vi "Comparison of the K-Means and MiniBatchKMeans clustering.vi"() -> ()   [LabVIEW 2020]
doc: "We want to compare the performance of the MiniBatchKMeans and KMeans: the MiniBatchKMeans is faster, but gives slightly different results.\n\nWe will cluster a set of data, first with KMeans and then with MiniBatchKMeans, and plot the results. We will also plot the points that are labelled differently between the two algorithms."
uses:
  Model/Unsupervised/Cluster/KMeans/Controls/kmeans_params.ctl
  Model/Unsupervised/Cluster/MiniBatchKMeans/Controls/mini_batch_kmeans_params.ctl
  PLAIYDISPLAY/Display/Classification/2D/Predicted/Controls/PredictedParameter.ctl
  PLAIYDISPLAY/Display/_Controls/Style.ctl
  Model/Unsupervised/Cluster/KMeans/KMeans.lvclass
  C:/Users/cipop/TDF Dropbox/2_Technologies de France/1 - Services et Etudes/PLAIY/2 - DEV/PLAIYLAB/code/Model/Model.lvclass
  Model/Unsupervised/Cluster/MiniBatchKMeans/MiniBatchKMeans.lvclass
  Model/Unsupervised/Cluster/KMeans/KMeans.vi
  Model/Unsupervised/Cluster/MiniBatchKMeans/MiniBatchKMeans.vi
  Preproc/Objet/6 - Datasets Transformation/6.8 - Pairwise metrics, Affinities and Kernels/Pairwise_distances_argmin/Pairwise_Distances_Argmin.vi
panel:
  in  "error in (no error)":errorcluster caption="entrée d'erreur (pas d'erreur)"
  in  "Local":T1
  out "identic":bool[](array[boolean])
  out "different":bool[](array[boolean])
  out "n_clusters":i32
  out "Plot 3":cluster{"X":dbl[], "Y":dbl[]}[](graph) caption="Difference"
  out "Plot 2":cluster{"X":dbl[], "Y":dbl[]}[](graph) caption="MiniBatchKMeans"
  out "error out":errorcluster
  out "Plot":cluster{"X":dbl[], "Y":dbl[]}[](graph) caption="KMeans"
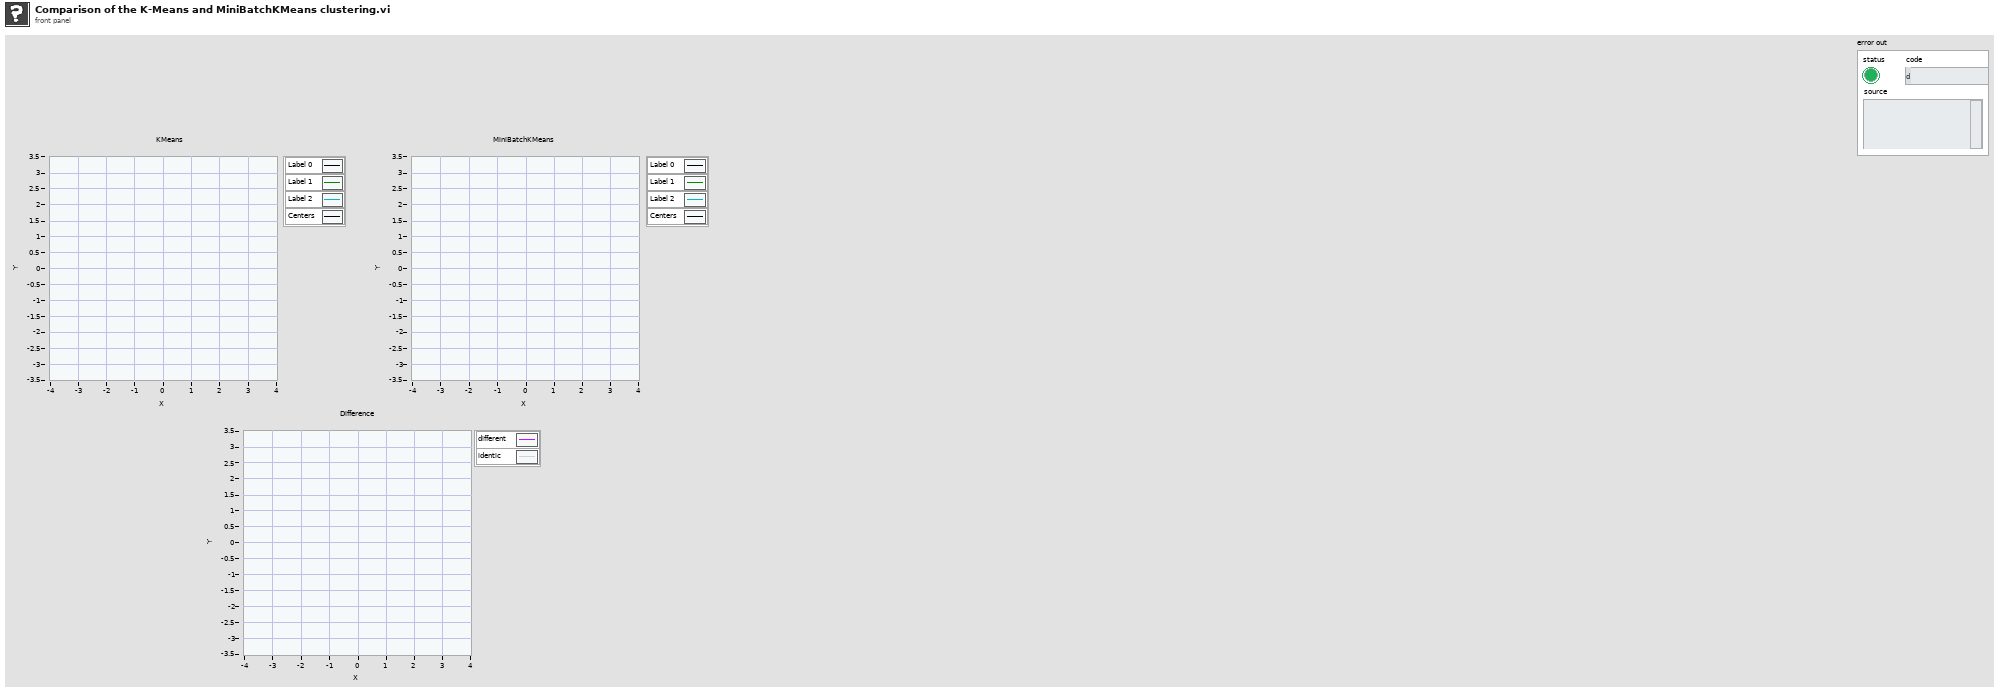
[diagram p1: front panel]
types:
  T1 = cluster{"X":dbl[][], "k_means_cluster_centers":dbl[][], "mbk.cluster_centers_":dbl[][], "k_means_labels":dbl[], "mbk_means_labels":dbl[], "order":dbl[], "mbk_means_cluster_centers":dbl[][]}
  T2 = cluster{"n_samples":i32[], "n_features":u32, "centers":i32[][], "cluster_std":dbl[], "centermin":dbl, "centermax":dbl, "shuffle":bool, "random_state":i32, "Returns":string}
  T3 = typedef "kmeans_params.ctl" = cluster{"n_clusters":dbl, "init":cluster{"init_type":string, "init_list":dbl[][]}, "n_init":dbl, "max_iter":dbl, "tol":dbl, "verbose":dbl, "random_state":dbl, "copy_x":bool, "algorithm":string}
  T4 = typedef "mini_batch_kmeans_params.ctl" = cluster{"n_clusters":dbl, "init":cluster{"init_type":string, "init_list":dbl[][]}, "max_iter":dbl, "batch_size":dbl, "verbose":dbl, "compute_labels":bool, "random_state":dbl, "tol":dbl, "max_no_improvement":dbl, "init_size":cluster{"init_size_type":string, "init_size_int":dbl}, "n_init":dbl, "reassignment_ratio":dbl}
  T5 = typedef "Style.ctl" = enum16{"Empty circle", "Full circle", "Empty square", "Full square", "Cross"}
  T6 = typedef "PredictedParameter.ctl" = cluster{"Plot":refnum<vi>, "Data":cluster{"X":dbl[][], "Predict":dbl[][]}, "Indexe":cluster{"X":i32, "Y":i32}, "Point Property":cluster{"Style":T5, "Label Color":u32[]}}
  T7 = cluster{" 4DArray":cluster{"1":string[][], "2":string[][]}[], " 3DArray":cluster{"Tableau":string[][]}[], "Sparse Matrix 2DArray":string[][], " 2DArray":string[][], " 1DArray":string[]}
  T8 = typedef "kmeans_attributes.ctl" = cluster{"cluster_centers_":dbl[][], "labels_":dbl[], "inertia_":dbl, "n_iter_":dbl}
  T9 = typedef "mini_batch_kmeans_attributes.ctl" = cluster{"cluster_centers_":dbl[][], "labels_":dbl[], "inertia_":dbl, "n_iter_":dbl}
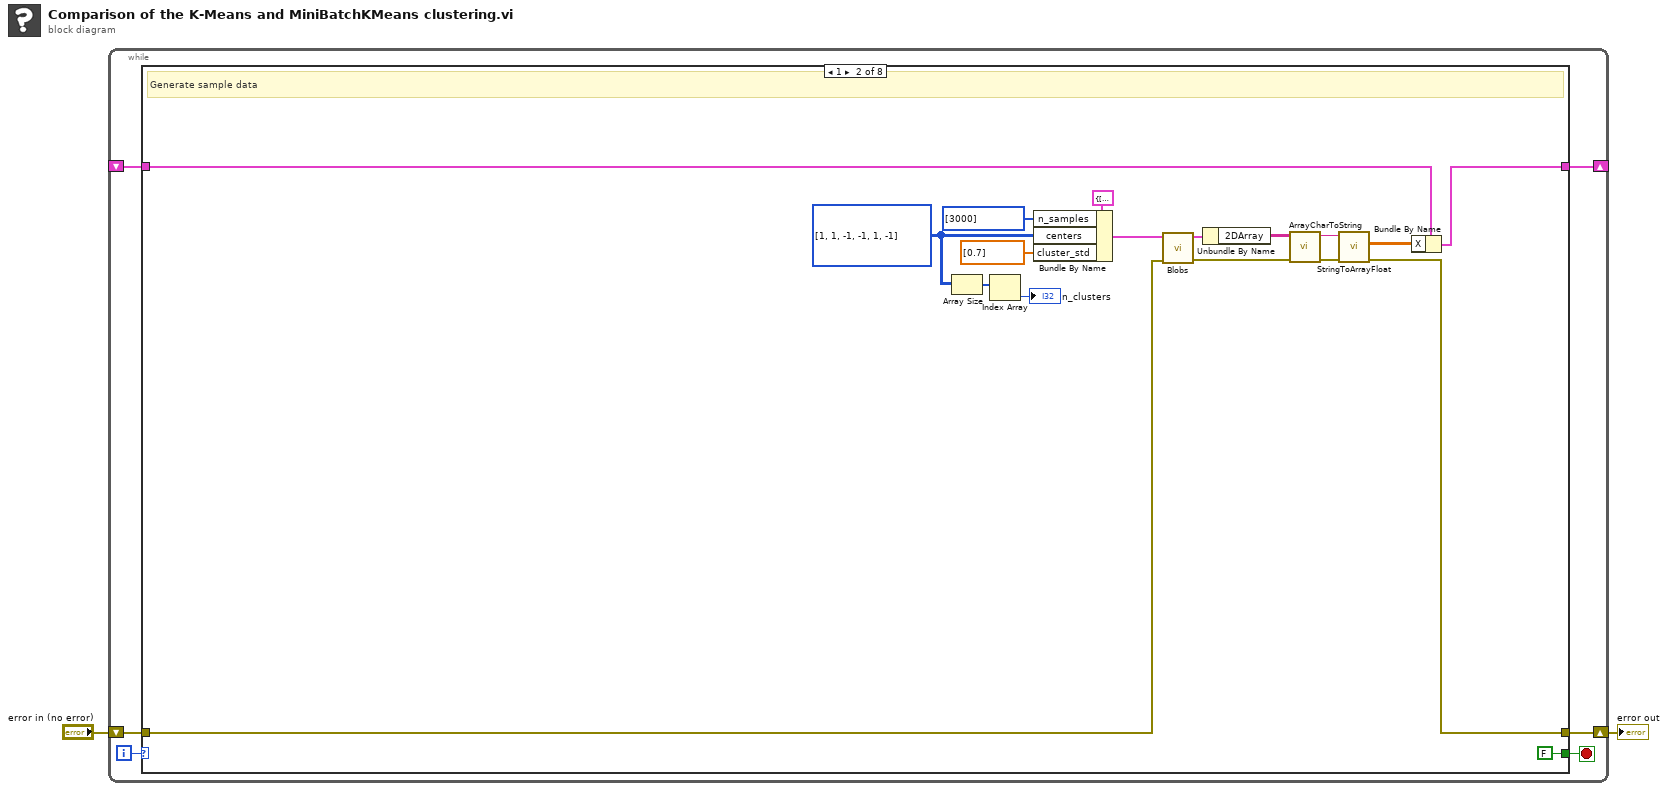
[diagram p0: block diagram]
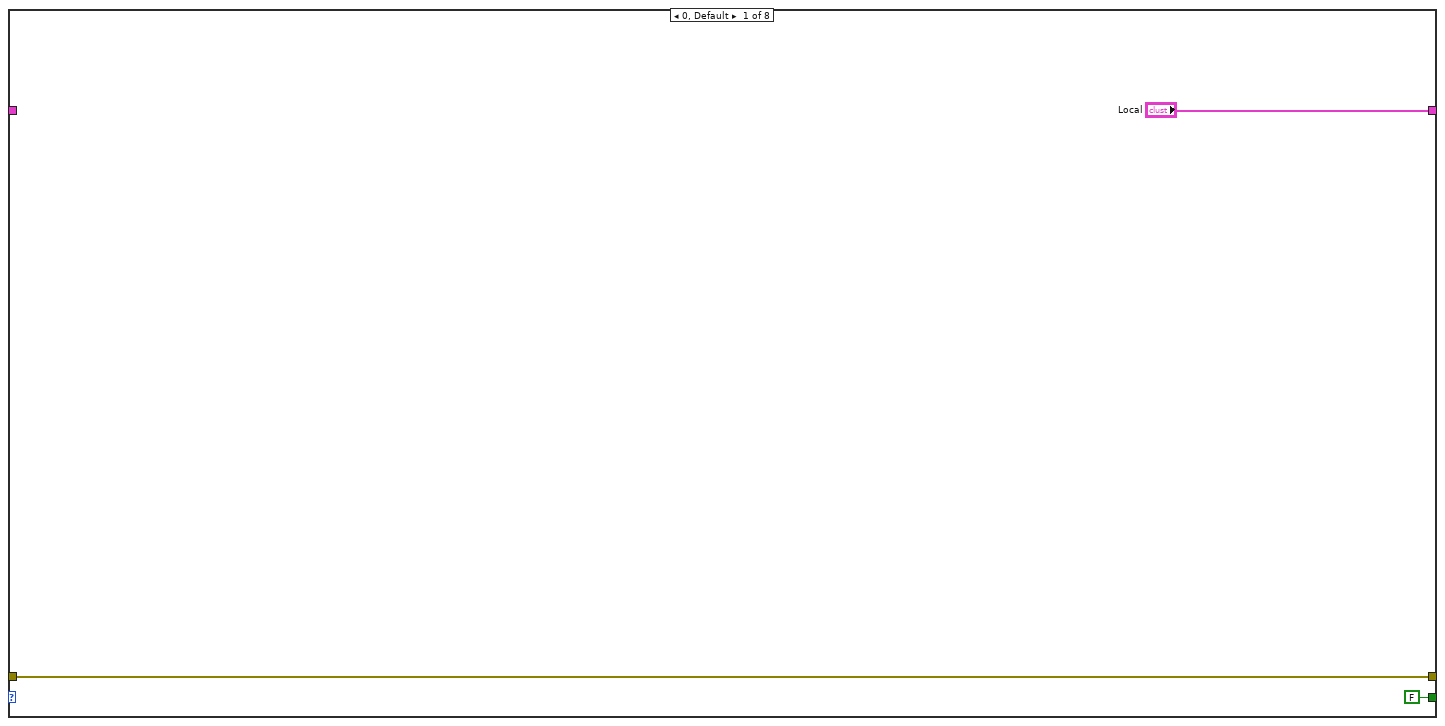
[diagram p2: hidden frame]
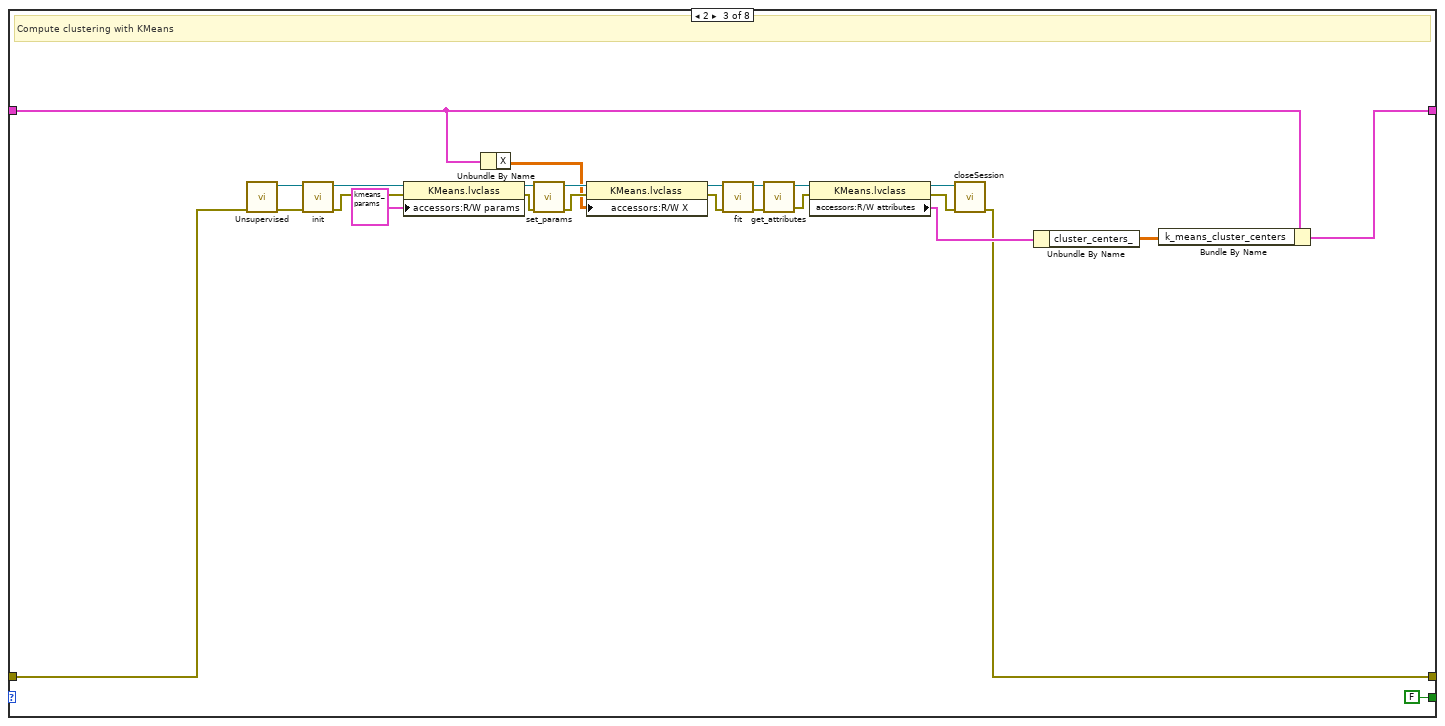
[diagram p3: hidden frame]
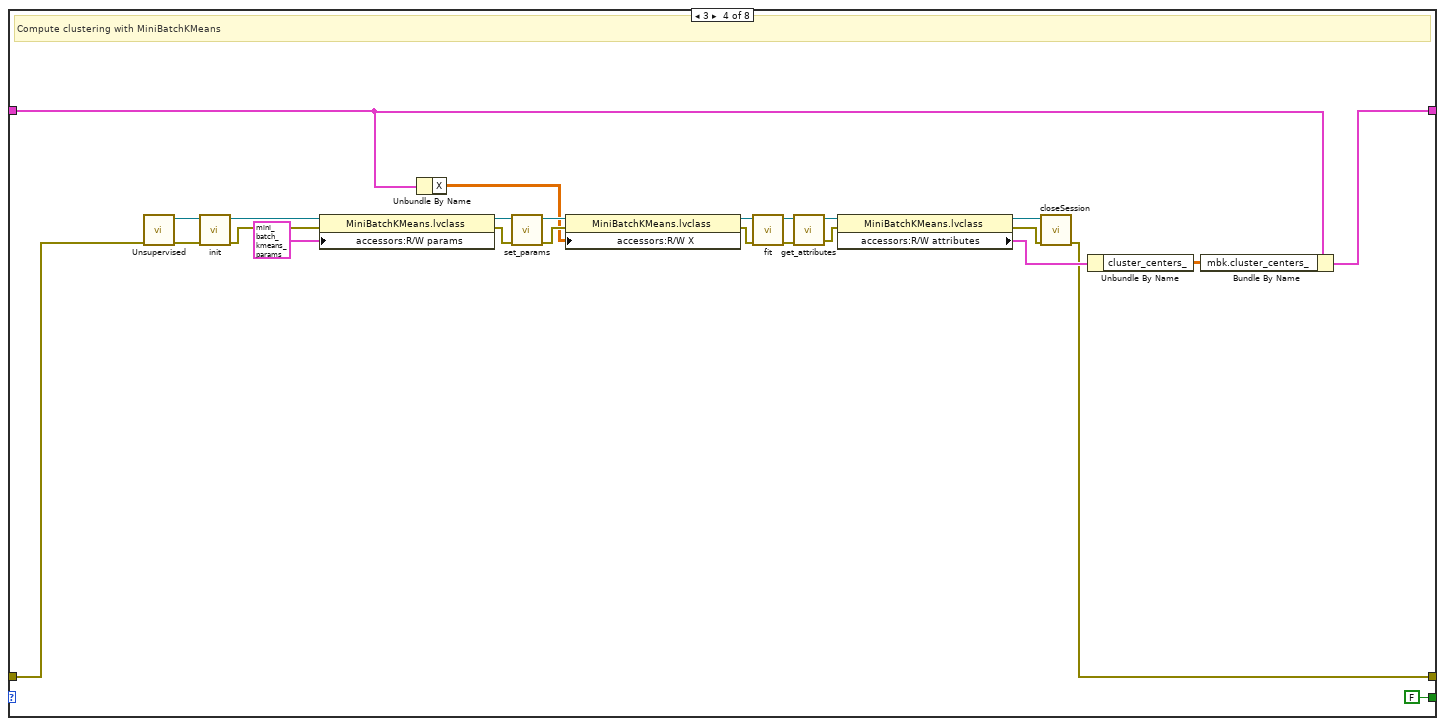
[diagram p4: hidden frame]
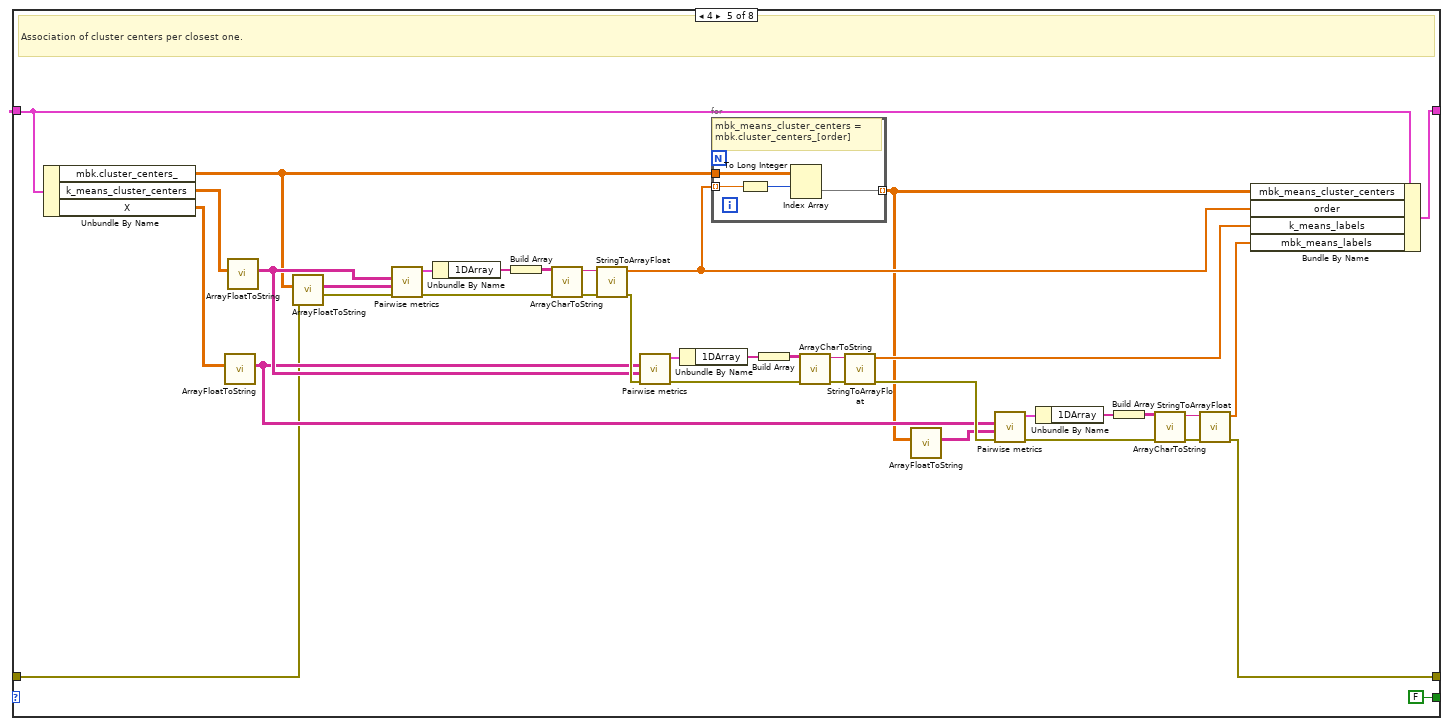
[diagram p5: hidden frame]
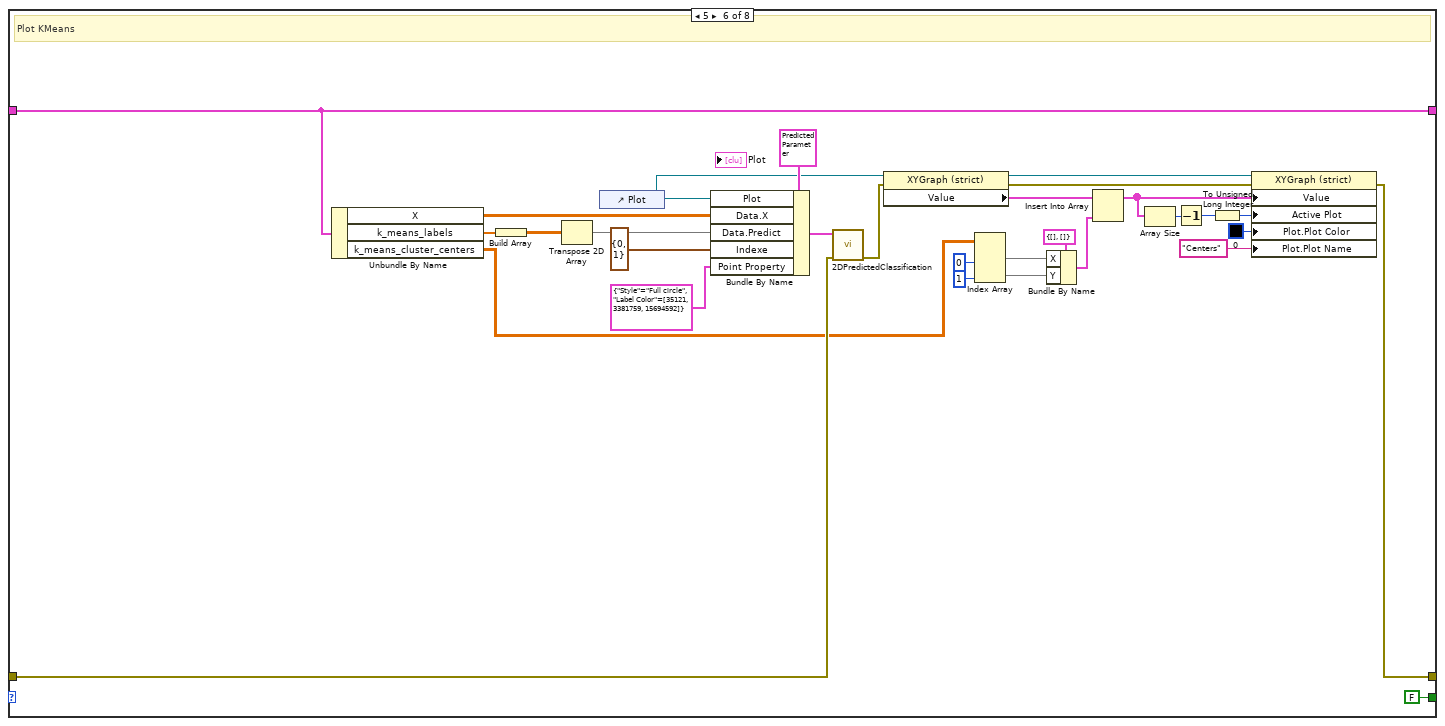
[diagram p6: hidden frame]
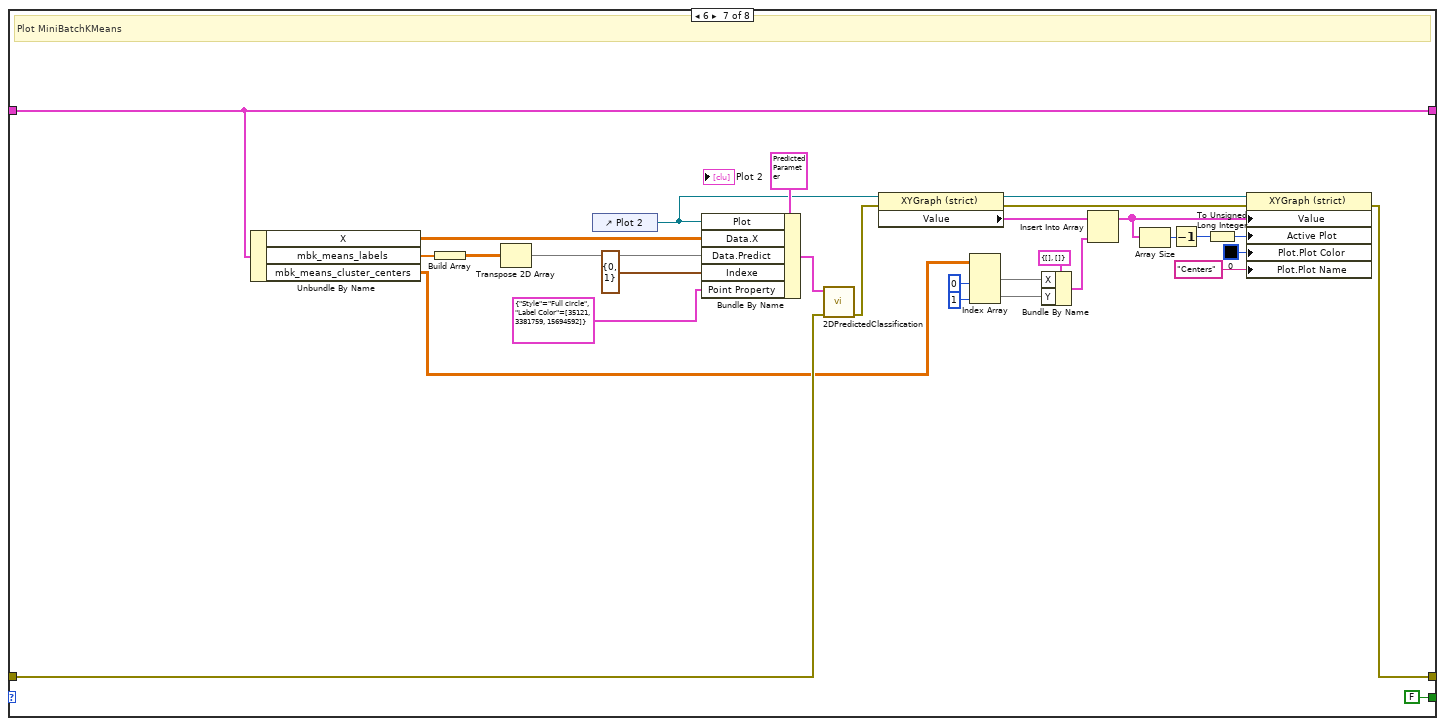
[diagram p7: hidden frame]
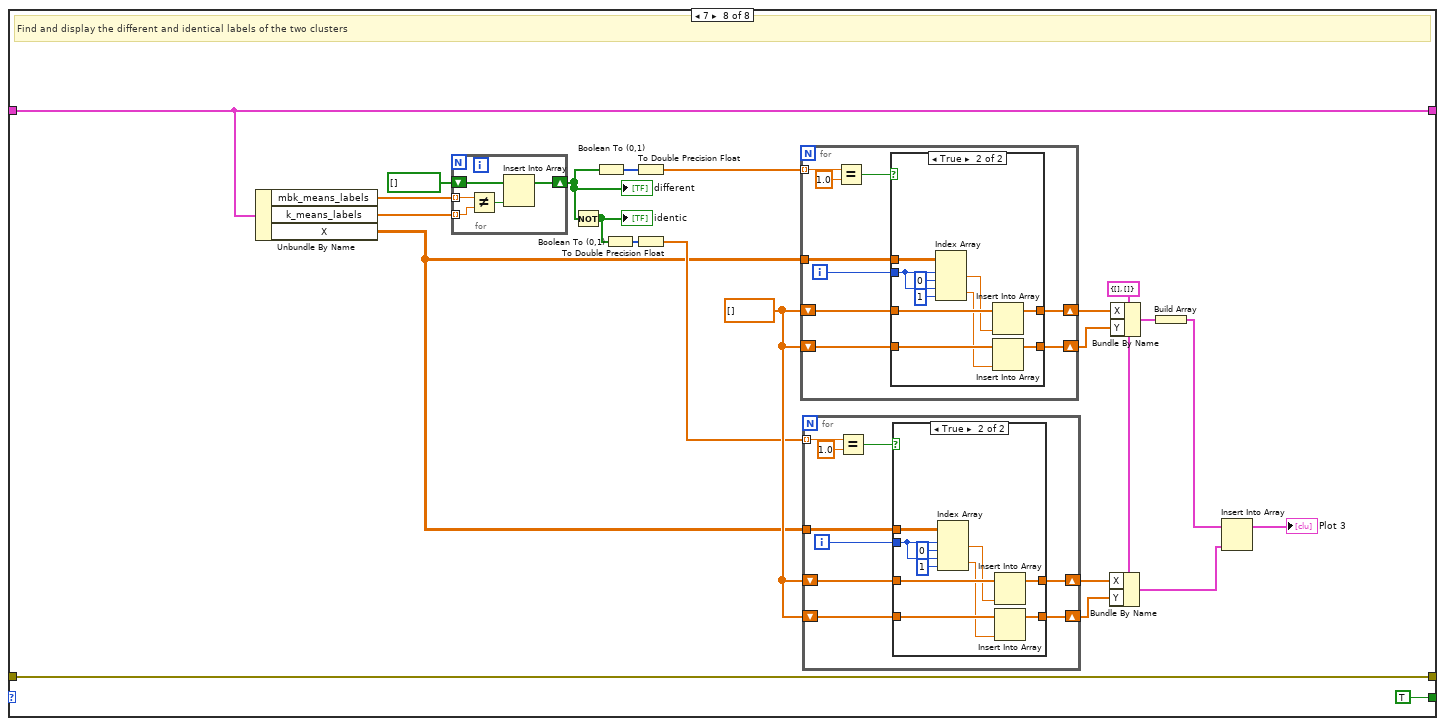
[diagram p8: hidden frame]
diagram:
  n1 = while {
    shift-right: [w7] -> _
    shift-left: _ -> [w6]
    shift-right: [w4] -> w1
    shift-left: "error in (no error)" -> [w5]
    i -> [w8]
    stop <- w3 stop-if-true
    n2 = case shown="1" w8 {
      tunnel: ["Local" w16 w33 w58 w85 w117 w150 w183] -> w7
      tunnel: w6 -> [_ w17 w34 w59 w80 w117 w150 w183]
      tunnel: w5 -> [w10 w14 w36 w55 w88 w123 w151 w177]
      tunnel: [w10 w13 w31 w56 w89 w124 w152 w177] -> w4
      tunnel: [FALSE FALSE FALSE FALSE FALSE FALSE FALSE TRUE] -> w3
      frame 0, Default {
      }
      frame 1 {
        w21 = i32[][] [[1, 1], [-1, -1], [1, -1]] ("centers")
        # "Generate sample data"
        n3 = Array Size(array=w21) -> (size(s)=w20:i32[])
        n4 = Index Array(array=w20) -> (element=→"n_clusters":i32)  [unwired: 1 in]
        n5 = Bundle By Name(cluster=T2 {"n_samples"=[100], "n_features"=2, "centers"=[], "cluster_std"=[1.0], "centermin"=-10.0, "centermax"=10.0, "shuffle"=TRUE, "random_state"=-1, "Returns"="X"} ("make_blobs"), "n_samples"=i32[] [3000], "centers"=w21, "cluster_std"=dbl[] [0.7]) -> (w22:T2)
        n6 = call "Blobs.vi"("error in (no error)"=w14, "make_blobs"=w22) -> ("error out"=w19:errorcluster, "Data"=w26:T7)  [unwired: 8 in]
        n7 = Unbundle By Name(w26) -> ("2DArray"=w27:string[][])
        n8 = call "ArrayCharToString.vi"("TAB"=w27) -> ("Instruction"=w28:string)  [unwired: 10 in]
        n9 = call "StringToArrayFloat.vi"("entrée d'erreur (pas d'erreur)"=w19, "Return value"=w28) -> ("error IO"=w13:errorcluster, "2DArray"=w15:dbl[][])  [unwired: 7 in, 1 out]
        n10 = Bundle By Name(cluster=w17, "X"=w15) -> (w16:T1)
      }
      frame 2 {
        # "Compute clustering with KMeans"
        n11 = call-poly "Unsupervised.vi"("error in"=w36) -> ("error out"=w41:errorcluster, "out"=w42:refnum<class "KMeans.lvclass">)  [unwired: 9 in]
        n12 = call-dynamic "init.vi"("error in (no error)"=w41, "Model en entrée"=w42) -> ("error out"=w47:errorcluster, "Model en sortie"=w51:refnum<class "KMeans.lvclass">)  [unwired: 8 in]
        n13 = property class="KMeans.lvclass"(reference=w51, error in=w47, "accessors:R/W params"=T3 {"n_clusters"=3.0, "init"={"init_type"="k-means++", "init_list"=[]}, "n_init"=10.0, "max_iter"=300.0, "tol"=0.0001, "verbose"=0.0, "random_state"=0.0, "copy_x"=TRUE, "algorithm"="auto"} ("KMeans params")) -> (reference out=w50:refnum<class "KMeans.lvclass">, error out=w40:errorcluster)
        n14 = Unbundle By Name(w34) -> ("X"=w35:dbl[][])
        n15 = call-dynamic "set_params.vi"("error in (no error)"=w40, "KMeans.lvclass 2"=w50) -> ("error out"=w48:errorcluster, "KMeans.lvclass"=w49:refnum<class "KMeans.lvclass">)  [unwired: 8 in]
        n16 = property class="KMeans.lvclass"(reference=w49, error in=w48, "accessors:R/W X"=w35) -> (reference out=w53:refnum<class "KMeans.lvclass">, error out=w52:errorcluster)
        n17 = call-dynamic "fit.vi"("error in (no error)"=w52, "KMeans.lvclass 2"=w53) -> ("error out"=w44:errorcluster, "KMeans.lvclass"=w45:refnum<class "KMeans.lvclass">)  [unwired: 8 in]
        n18 = call-dynamic "get_attributes.vi"("error in (no error)"=w44, "KMeans.lvclass 2"=w45) -> ("error out"=w37:errorcluster, "KMeans.lvclass"=w38:refnum<class "KMeans.lvclass">)  [unwired: 8 in]
        n19 = property class="KMeans.lvclass"(reference=w38, error in=w37) -> (reference out=w46:refnum<class "KMeans.lvclass">, error out=w39:errorcluster, "accessors:R/W attributes"=w43:T8)
        n20 = call-dynamic "closeSession.vi"("error in"=w39, "Python en entrée"=w46) -> ("error out"=w31:errorcluster)  [unwired: 8 in, 1 out]
        n21 = Unbundle By Name(w43) -> ("cluster_centers_"=w32:dbl[][])
        n22 = Bundle By Name(cluster=w34, "k_means_cluster_centers"=w32) -> (w33:T1)
      }
      frame 3 {
        # "Compute clustering with MiniBatchKMeans"
        n23 = call-poly "Unsupervised.vi"("error in"=w55) -> ("error out"=w78:errorcluster, "out"=w77:refnum<class "MiniBatchKMeans.lvclass">)  [unwired: 9 in]
        n24 = call-dynamic "init.vi"("error in (no error)"=w78, "Model en entrée"=w77) -> ("error out"=w75:errorcluster, "Model en sortie"=w72:refnum<class "MiniBatchKMeans.lvclass">)  [unwired: 8 in]
        n25 = property class="MiniBatchKMeans.lvclass"(reference=w72, error in=w75, "accessors:R/W params"=T4 {"n_clusters"=3.0, "init"={"init_type"="k-means++", "init_list"=[]}, "max_iter"=100.0, "batch_size"=45.0, "verbose"=0.0, "compute_labels"=TRUE, "random_state"=0.0, "tol"=0.0, "max_no_improvement"=10.0, "init_size"={"init_size_type"="None", "init_size_int"=0.0}, "n_init"=10.0, "reassignment_ratio"=0.01} ("MiniBatchKMeans params")) -> (reference out=w73:refnum<class "MiniBatchKMeans.lvclass">, error out=w69:errorcluster)
        n26 = Unbundle By Name(w59) -> ("X"=w60:dbl[][])
        n27 = call-dynamic "set_params.vi"("error in (no error)"=w69, "MiniBatchKMeans.lvclass 2"=w73) -> ("error out"=w68:errorcluster, "MiniBatchKMeans.lvclass"=w74:refnum<class "MiniBatchKMeans.lvclass">)  [unwired: 8 in]
        n28 = property class="MiniBatchKMeans.lvclass"(reference=w74, error in=w68, "accessors:R/W X"=w60) -> (reference out=w71:refnum<class "MiniBatchKMeans.lvclass">, error out=w67:errorcluster)
        n29 = call-dynamic "fit.vi"("error in (no error)"=w67, "MiniBatchKMeans.lvclass 2"=w71) -> ("error out"=w63:errorcluster, "MiniBatchKMeans.lvclass"=w64:refnum<class "MiniBatchKMeans.lvclass">)  [unwired: 8 in]
        n30 = call-dynamic "get_attributes.vi"("error in (no error)"=w63, "MiniBatchKMeans.lvclass 2"=w64) -> ("error out"=w61:errorcluster, "MiniBatchKMeans.lvclass"=w62:refnum<class "MiniBatchKMeans.lvclass">)  [unwired: 8 in]
        n31 = property class="MiniBatchKMeans.lvclass"(reference=w62, error in=w61) -> (reference out=w76:refnum<class "MiniBatchKMeans.lvclass">, error out=w66:errorcluster, "accessors:R/W attributes"=w65:T9)
        n32 = call-dynamic "closeSession.vi"("error in"=w66, "Python en entrée"=w76) -> ("error out"=w56:errorcluster)  [unwired: 8 in, 1 out]
        n33 = Unbundle By Name(w65) -> ("cluster_centers_"=w57:dbl[][])
        n34 = Bundle By Name(cluster=w59, "mbk.cluster_centers_"=w57) -> (w58:T1)
      }
      frame 4 {
        # "Association of cluster centers per closest one."
        n35 = Unbundle By Name(w80) -> ("mbk.cluster_centers_"=w90:dbl[][], "k_means_cluster_centers"=w87:dbl[][], "X"=w86:dbl[][])
        n36 = call "ArrayFloatToString.vi"("2D Data"=w86) -> ("Array"=w92:string[][])  [unwired: 9 in, 1 out]
        n37 = call "ArrayFloatToString.vi"("2D Data"=w87) -> ("Array"=w99:string[][])  [unwired: 9 in, 1 out]
        n38 = call "ArrayFloatToString.vi"("2D Data"=w90) -> ("Array"=w111:string[][])  [unwired: 9 in, 1 out]
        n39 = call-poly "Pairwise metrics.vi"("error in"=w88, "Y"=w111, "X"=w99) -> ("error out"=w109:errorcluster, "Data"=w110:T7)  [unwired: 7 in]
        n40 = Unbundle By Name(w110) -> ("1DArray"=w107:string[])
        n41 = Build Array(w107) -> (w106:string[][])
        n42 = call "ArrayCharToString.vi"("TAB"=w106) -> ("Instruction"=w108:string)  [unwired: 10 in]
        n43 = call "StringToArrayFloat.vi"("entrée d'erreur (pas d'erreur)"=w109, "Return value"=w108) -> ("error IO"=w100:errorcluster, "1DArray"=w82:dbl[])  [unwired: 7 in, 1 out]
        n44 = call-poly "Pairwise metrics.vi"("error in"=w100, "Y"=w99, "X"=w92) -> ("error out"=w102:errorcluster, "Data"=w101:T7)  [unwired: 7 in]
        n45 = Unbundle By Name(w101) -> ("1DArray"=w104:string[])
        n46 = for {
          tunnel: w82 -> [w114] mode=indexing
          tunnel: w90 -> [w115]
          tunnel: [w113] -> w81 mode=indexing
          # "mbk_means_cluster_centers = mbk.cluster_centers_[order]"
          n47 = To Long Integer(number=w114) -> (32bit integer=w112:i32)
          n48 = Index Array(array=w115, index (row)=w112) -> (element=w113:dbl[])  [unwired: 1 in]
        }
        n49 = Build Array(w104) -> (w105:string[][])
        n50 = call "ArrayCharToString.vi"("TAB"=w105) -> ("Instruction"=w103:string)  [unwired: 10 in]
        n51 = call "StringToArrayFloat.vi"("entrée d'erreur (pas d'erreur)"=w102, "Return value"=w103) -> ("error IO"=w93:errorcluster, "1DArray"=w84:dbl[])  [unwired: 7 in, 1 out]
        n52 = call "ArrayFloatToString.vi"("2D Data"=w81) -> ("Array"=w91:string[][])  [unwired: 9 in, 1 out]
        n53 = call-poly "Pairwise metrics.vi"("error in"=w93, "Y"=w91, "X"=w92) -> ("error out"=w97:errorcluster, "Data"=w98:T7)  [unwired: 7 in]
        n54 = Unbundle By Name(w98) -> ("1DArray"=w95:string[])
        n55 = Build Array(w95) -> (w94:string[][])
        n56 = call "ArrayCharToString.vi"("TAB"=w94) -> ("Instruction"=w96:string)  [unwired: 10 in]
        n57 = call "StringToArrayFloat.vi"("entrée d'erreur (pas d'erreur)"=w97, "Return value"=w96) -> ("error IO"=w89:errorcluster, "1DArray"=w83:dbl[])  [unwired: 7 in, 1 out]
        n58 = Bundle By Name(cluster=w80, "mbk_means_cluster_centers"=w81, "order"=w82, "k_means_labels"=w84, "mbk_means_labels"=w83) -> (w85:T1)
      }
      frame 5 {
        # "Plot KMeans"
        n59 = Unbundle By Name(w117) -> ("X"=w122:dbl[][], "k_means_labels"=w120:dbl[], "k_means_cluster_centers"=w118:dbl[][])
        n60 = Build Array(w120) -> (w121:dbl[][])
        n61 = Transpose 2D Array(2D array=w121) -> (transposed array=w119:dbl[][])
        n62 = control-ref of="Plot"() -> (w125:refnum<vi>)
        n63 = Bundle By Name(cluster=T6 {"Plot"=refnum, "Data"={"X"=[], "Predict"=[]}, "Indexe"={"X"=0, "Y"=1}, "Point Property"={"Style"=enum."Full circle", "Label Color"=[8978528, 4367871, 1985280]}} ("Parameters"), "Plot"=w125, "Data.X"=w122, "Data.Predict"=w119, "Indexe"=cluster{"X":i32, "Y":i32} {"X"=0, "Y"=1}, "Point Property"=cluster{"Style":T5, "Label Color":u32[]} {"Style"=enum."Full circle", "Label Color"=[35121, 3381759, 15694592]}) -> (w144:T6)
        n64 = call "2DPredictedClassification.vi"("error in"=w123, "Parameters"=w144) -> ("error out"=w134:errorcluster)  [unwired: 9 in]
        n65 = property class="XYGraph (strict)"(reference=w125, error in=w134) -> (reference out=w127:refnum<vi>, error out=w133:errorcluster, "Value"=w141:cluster{"X":dbl[], "Y":dbl[]}[])
        n66 = Index Array(array=w118, index (col) #1=0 ("disabled index (col)"), index (col) #2=1 ("index (col)")) -> (element #1=w139:dbl[], element #2=w135:dbl[])  [unwired: 2 in]
        n67 = Bundle By Name(cluster=cluster{"X":dbl[], "Y":dbl[]} {"X"=[], "Y"=[]} ("new element/subarray"), "X"=w139, "Y"=w135) -> (w138:cluster{"X":dbl[], "Y":dbl[]})
        n68 = Insert Into Array(array=w141, new element=w138) -> (w128:cluster{"X":dbl[], "Y":dbl[]}[])  [unwired: 1 in]
        n69 = Array Size(array=w128) -> (size(s)=w132:i32)
        n70 = Decrement(x=w132) -> (x-1=w126:i32)
        n71 = To Unsigned Long Integer(number=w126) -> (unsigned 32bit integer=w130:u32)
        n72 = property class="XYGraph (strict)"(reference=w127, error in=w133, "Value"=w128, "Active Plot"=w130, "Plot.Plot Color"=u32 0, "Plot.Plot Name"="Centers") -> (error out=w124:errorcluster)  [unwired: 1 out]
      }
      frame 6 {
        # "Plot MiniBatchKMeans"
        n73 = Unbundle By Name(w150) -> ("X"=w149:dbl[][], "mbk_means_labels"=w148:dbl[], "mbk_means_cluster_centers"=w147:dbl[][])
        n74 = Build Array(w148) -> (w171:dbl[][])
        n75 = Transpose 2D Array(2D array=w171) -> (transposed array=w170:dbl[][])
        n76 = control-ref of="Plot 2"() -> (w153:refnum<vi>)
        n77 = Bundle By Name(cluster=T6 {"Plot"=refnum, "Data"={"X"=[], "Predict"=[]}, "Indexe"={"X"=0, "Y"=1}, "Point Property"={"Style"=enum."Full circle", "Label Color"=[8978528, 4367871, 1985280]}} ("Parameters"), "Plot"=w153, "Data.X"=w149, "Data.Predict"=w170, "Indexe"=cluster{"X":i32, "Y":i32} {"X"=0, "Y"=1}, "Point Property"=cluster{"Style":T5, "Label Color":u32[]} {"Style"=enum."Full circle", "Label Color"=[35121, 3381759, 15694592]}) -> (w173:T6)
        n78 = call "2DPredictedClassification.vi"("error in"=w151, "Parameters"=w173) -> ("error out"=w154:errorcluster)  [unwired: 9 in]
        n79 = property class="XYGraph (strict)"(reference=w153, error in=w154) -> (reference out=w168:refnum<vi>, error out=w162:errorcluster, "Value"=w155:cluster{"X":dbl[], "Y":dbl[]}[])
        n80 = Index Array(array=w147, index (col) #1=0 ("disabled index (col)"), index (col) #2=1 ("index (col)")) -> (element #1=w157:dbl[], element #2=w161:dbl[])  [unwired: 2 in]
        n81 = Bundle By Name(cluster=cluster{"X":dbl[], "Y":dbl[]} {"X"=[], "Y"=[]} ("new element/subarray"), "X"=w157, "Y"=w161) -> (w158:cluster{"X":dbl[], "Y":dbl[]})
        n82 = Insert Into Array(array=w155, new element=w158) -> (w167:cluster{"X":dbl[], "Y":dbl[]}[])  [unwired: 1 in]
        n83 = Array Size(array=w167) -> (size(s)=w163:i32)
        n84 = Decrement(x=w163) -> (x-1=w169:i32)
        n85 = To Unsigned Long Integer(number=w169) -> (unsigned 32bit integer=w165:u32)
        n86 = property class="XYGraph (strict)"(reference=w168, error in=w162, "Value"=w167, "Active Plot"=w165, "Plot.Plot Color"=u32 0, "Plot.Plot Name"="Centers") -> (error out=w152:errorcluster)  [unwired: 1 out]
      }
      frame 7 {
        w187 = cluster{"X":dbl[], "Y":dbl[]} {"X"=[], "Y"=[]} ("new element/subarray")
        w191 = dbl[] [] ("1DArray")
        # "Find and display the different and identical labels of the two clusters"
        n87 = Unbundle By Name(w183) -> ("mbk_means_labels"=w182:dbl[], "k_means_labels"=w181:dbl[], "X"=w180:dbl[][])
        n88 = for {
          tunnel: w182 -> [w242] mode=indexing
          tunnel: w181 -> [w241] mode=indexing
          shift-right: [w243] -> w179
          shift-left: bool[] [] -> [w245]
          n89 = Not Equal?(x=w242, y=w241) -> (x != y?=w244:bool)
          n90 = Insert Into Array(array=w245, new element=w244) -> (w243:bool[])  [unwired: 1 in]
        }
        "different" <- w179
        n91 = Not(x=w179) -> (.not. x?=w178:bool[])
        "identic" <- w178
        n92 = Boolean To (0,1)(Boolean=w179) -> (0, 1=w197:i16[])
        n93 = Boolean To (0,1)(Boolean=w178) -> (0, 1=w196:i16[])
        n94 = To Double Precision Float(number=w197) -> (double precision float=w195:dbl[])
        n95 = To Double Precision Float(number=w196) -> (double precision float=w190:dbl[])
        n96 = for {
          tunnel: w195 -> [w228] mode=indexing
          tunnel: w180 -> [w225]
          shift-right: [w222] -> w194
          shift-left: w191 -> [w223]
          shift-right: [w220] -> w193
          shift-left: w191 -> [w221]
          i -> [w224]
          n97 = Equal?(x=w228, y=1.0) -> (x = y?=w226:bool)
          n98 = case shown="True" w226 {
            tunnel: w225 -> [_ w240]
            tunnel: w224 -> [_ w237]
            tunnel: w223 -> [w230 w236]
            tunnel: [w230 w234] -> w222
            tunnel: w221 -> [w229 w233]
            tunnel: [w229 w231] -> w220
            frame False {
            }
            frame True {
              n99 = Index Array(array=w240, index (row) #1=w237, index (col) #1=0 ("disabled index (col)"), index (row) #2=w237, index (col) #2=1 ("index (col)")) -> (element #1=w235:dbl, element #2=w232:dbl)
              n100 = Insert Into Array(array=w236, new element=w235) -> (w234:dbl[])  [unwired: 1 in]
              n101 = Insert Into Array(array=w233, new element=w232) -> (w231:dbl[])  [unwired: 1 in]
            }
          }
        }
        n102 = for {
          tunnel: w190 -> [w207] mode=indexing
          tunnel: w180 -> [w199]
          shift-right: [w202] -> w189
          shift-left: w191 -> [w203]
          shift-right: [w200] -> w188
          shift-left: w191 -> [w201]
          i -> [w204]
          n103 = Equal?(x=w207, y=1.0) -> (x = y?=w205:bool)
          n104 = case shown="True" w205 {
            tunnel: w199 -> [_ w219]
            tunnel: w204 -> [_ w216]
            tunnel: w203 -> [w209 w215]
            tunnel: [w209 w213] -> w202
            tunnel: w201 -> [w208 w212]
            tunnel: [w208 w210] -> w200
            frame False {
            }
            frame True {
              n105 = Index Array(array=w219, index (row) #1=w216, index (col) #1=0 ("disabled index (col)"), index (row) #2=w216, index (col) #2=1 ("index (col)")) -> (element #1=w214:dbl, element #2=w211:dbl)
              n106 = Insert Into Array(array=w215, new element=w214) -> (w213:dbl[])  [unwired: 1 in]
              n107 = Insert Into Array(array=w212, new element=w211) -> (w210:dbl[])  [unwired: 1 in]
            }
          }
        }
        n108 = Bundle By Name(cluster=w187, "X"=w189, "Y"=w188) -> (w185:cluster{"X":dbl[], "Y":dbl[]})
        n109 = Bundle By Name(cluster=w187, "X"=w194, "Y"=w193) -> (w192:cluster{"X":dbl[], "Y":dbl[]})
        n110 = Build Array(w192) -> (w186:cluster{"X":dbl[], "Y":dbl[]}[])
        n111 = Insert Into Array(array=w186, new element=w185) -> (→"Plot 3":cluster{"X":dbl[], "Y":dbl[]}[])  [unwired: 1 in]
      }
    }
  }
  "error out" <- w1
